vi "note.vi"() -> ()   [LabVIEW 2018]
panel:
  out "test":dbl
  out "Note a faire 2":dbl
  in  "String 2":string
  out "String":string
  out "Note a faire":dbl
  in  "Moyenne visée":dbl=1.0 min=1.0 max=6.0 step=0.5
  out "Moyenne actuelle":dbl
  in  "Array":dbl[](array[numeric]) min=1.0 max=6.0 step=0.5
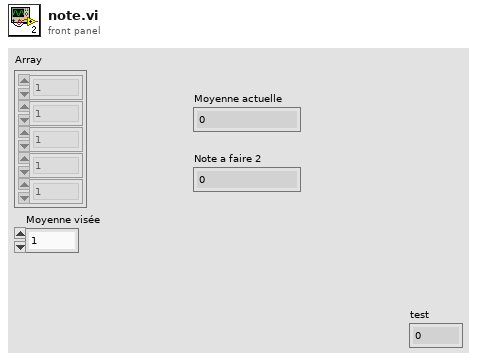
[diagram p1: front panel]
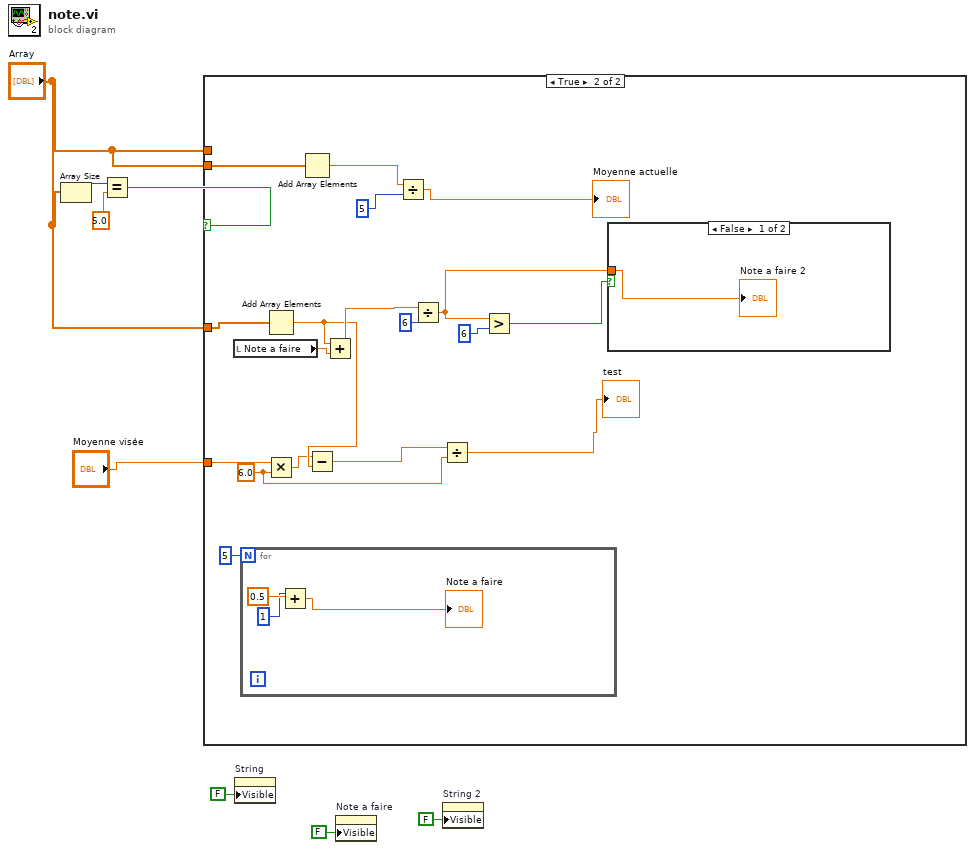
[diagram p0: block diagram]
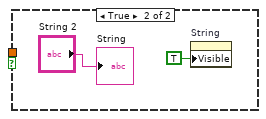
[diagram p3: hidden frame]
diagram:
  n1 = Array Size(array="Array") -> (size(s)=w6:i32)
  n2 = Equal?(x=w6, y=5.0) -> (x = y?=w7:bool)
  n3 = case shown="True" w7 {
    tunnel: "Array" -> [_ w24]
    tunnel: "Array" -> [_ _]
    tunnel: "Array" -> [_ w22]
    tunnel: "Moyenne visée" -> [_ w14]
    frame False {
    }
    frame True {
      w11 = 6.0 ("y")
      n4 = local read "Note a faire"() -> (w18:dbl)
      n5 = for {
        N: 5 -> [_]
        n6 = Add(x=1, y=0.5) -> (x+y=→"Note a faire":dbl)
      }
      n7 = Add Array Elements(numeric array=w22) -> (sum=w13:dbl)
      n8 = Multiply(x=w14, y=w11) -> (x*y=w12:dbl)
      n9 = Add Array Elements(numeric array=w24) -> (sum=w23:dbl)
      n10 = Subtract(x=w12, y=w13) -> (x-y=w10:dbl)
      n11 = Add(x=w13, y=w18) -> (x+y=w20:dbl)
      n12 = Divide(x=w23, y=5) -> (x/y=→"Moyenne actuelle":dbl)
      n13 = Divide(x=w20, y=6) -> (x/y=w15:dbl)
      n14 = Divide(x=w10, y=w11) -> (x/y=→"test":dbl)
      n15 = Greater?(x=w15, y=6) -> (0:w16:bool)
      n16 = case shown="False" w16 {
        tunnel: w15 -> [w27 _]
        frame False {
          "Note a faire 2" <- w27
        }
        frame True {
          n17 = property on="String" class="Str"("Visible"=TRUE) -> ()  [unwired: 2 in, 2 out]
          "String" <- "String 2"
        }
      }
    }
  }
  n18 = property on="String" class="Str"("Visible"=FALSE) -> ()  [unwired: 2 in, 2 out]
  n19 = property on="Note a faire" class="DigNum (strict)"("Visible"=FALSE) -> ()  [unwired: 2 in, 2 out]
  n20 = property on="String 2" class="Str"("Visible"=FALSE) -> ()  [unwired: 2 in, 2 out]
